vi "linear_activation_backward.vi"(3 "activation":enum16{"sigmoid", "relu"}(ring), 4 "linear_cache":cluster{"A":dbl[][], "W":dbl[][], "b":dbl[][]}, 5 "Z":dbl[][](array[numeric]), 6 "dA":dbl[][](array[numeric])) -> (0 "db":dbl[][](array[numeric]), 1 "dW":dbl[][](array[numeric]), 2 "dA_prev":dbl[][](array[numeric]))   [LabVIEW 2020]
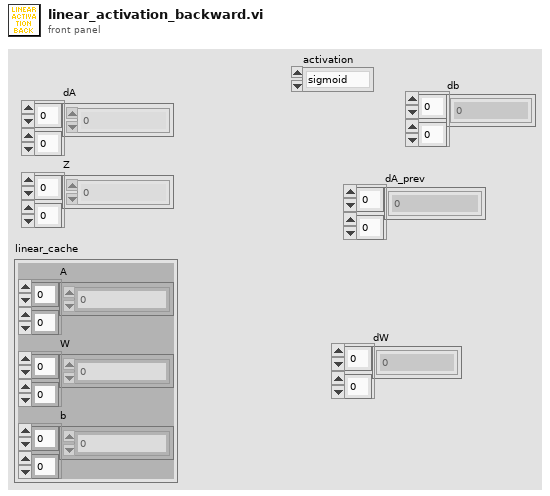
[diagram p1: front panel]
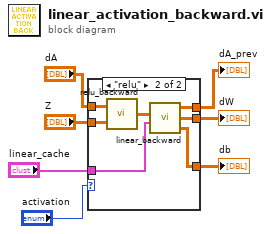
[diagram p0: block diagram]
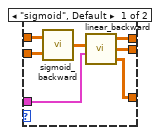
[diagram p2: hidden frame]
diagram:
  n1 = case shown="\"relu\"" "activation" {
    tunnel: "dA" -> [w14 w21]
    tunnel: "Z" -> [w13 w20]
    tunnel: "linear_cache" -> [w11 w18]
    tunnel: [w10 w17] -> w3
    tunnel: [w9 w16] -> w2
    tunnel: [w8 w15] -> w1
    frame "sigmoid", Default {
      n2 = call "sigmoid_backward.vi"("Z"=w13, "dA"=w14) -> ("dZ"=w12:dbl[][])
      n3 = call "linear_backward.vi"("cache"=w11, "dZ"=w12) -> ("db"=w8:dbl[][], "dW"=w9:dbl[][], "dA_prev"=w10:dbl[][])  [unwired: 2 in]
    }
    frame "relu" {
      n4 = call "relu_backward.vi"("Z"=w20, "dA"=w21) -> ("dZ"=w19:dbl[][])
      n5 = call "linear_backward.vi"("cache"=w18, "dZ"=w19) -> ("db"=w15:dbl[][], "dW"=w16:dbl[][], "dA_prev"=w17:dbl[][])  [unwired: 2 in]
    }
  }
  "dA_prev" <- w3
  "dW" <- w2
  "db" <- w1
